vi "3D Plot and Log File Trial1.vi"() -> ()   [LabVIEW 2013]
doc: "This example shows how to use the driver's VI's to set up the Polaris and acquire transformations. For this example, all wired tools are activated and one wireless tool is activated."
uses:
  <vilib>/Platform/NI_3dgraph.lvlib
panel:
  in  "Output File":path=path "c:/polaris.txt"
  in  "STOP 2":bool
  in  "Track Outside Measurement Volume? (F:No) 2":bool
  in  "Track Stray Markers? (F:No)":bool
  out "Current Transformations 2":T1(array[cluster])
  in  "Location of ROM File for Tool":path=path "C:/Program Files/Northern Digital Inc/8700248.rom"
  in  "Serial Configuration":T2={"Baud Rate (9600)"=9600, "Flow Control (0:None)"=0, "Parity"=0, "Data Bits"=8, "Stop Bits"=10} {"Stop Bits" items=["1.0"=10, "2.0"=20]; "Parity" items=["None", "Odd", "Even"]; "Flow Control (0:None)" items=["None", "XON/XOFF"]; "Baud Rate (9600)" items=["9600"=9600, "14.4k"=14400, "19.2k"=19200, "38.4k"=38400, "57.6k "=57600, "115.2k"=115200]}
  out "Current Transformations":T1(array[cluster])
  in  "VISA resource name":refnum<visa-resource-name>="COM1"
  in  "Reset? (T:Yes)":bool=TRUE
  in  "3D Curve":refnum<k7>(container)
  in  "Track Outside Measurement Volume? (F:No)":bool
  in  "Plot Data? (T:Yes)":bool=TRUE
  in  "STOP":bool
  # "NOTE: This VI will only run on machines using a Windows OS (for ActiveX support).  Plotting this 3D data\nis NOT meant for performance, rather it is intended to give a more intuitive representation of the data\nreturned by the Polaris instrument.  For demonstration of faster acquisition, please take a look at the\nndipolaris Measurement Exampole VI."
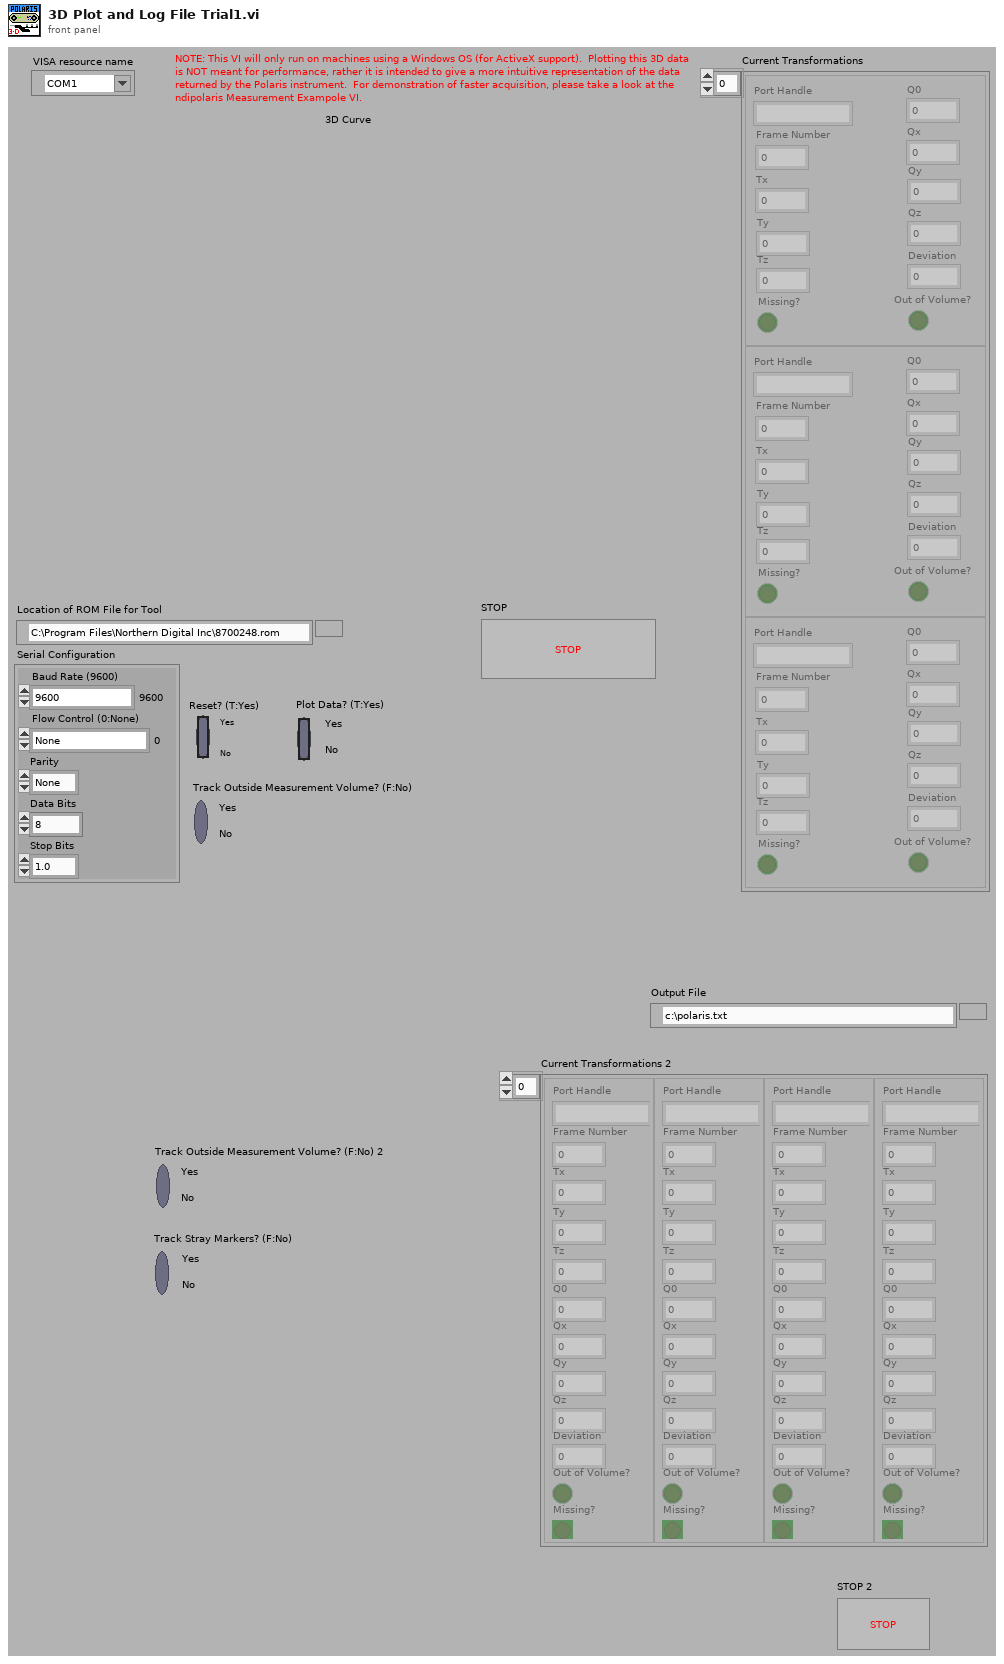
[diagram p1: front panel]
types:
  T1 = cluster{"Port Handle":string, "Frame Number":u32, "Tx":dbl, "Ty":dbl, "Tz":dbl, "Q0":dbl, "Qx":dbl, "Qy":dbl, "Qz":dbl, "Deviation":dbl, "Missing?":bool, "Out of Volume?":bool}[]
  T2 = cluster{"Baud Rate (9600)":u32, "Flow Control (0:None)":u16, "Parity":u16, "Data Bits":u16, "Stop Bits":u16}
  T3 = enum16{"open", "open or create", "create or replace", "create", "open (read only)"}
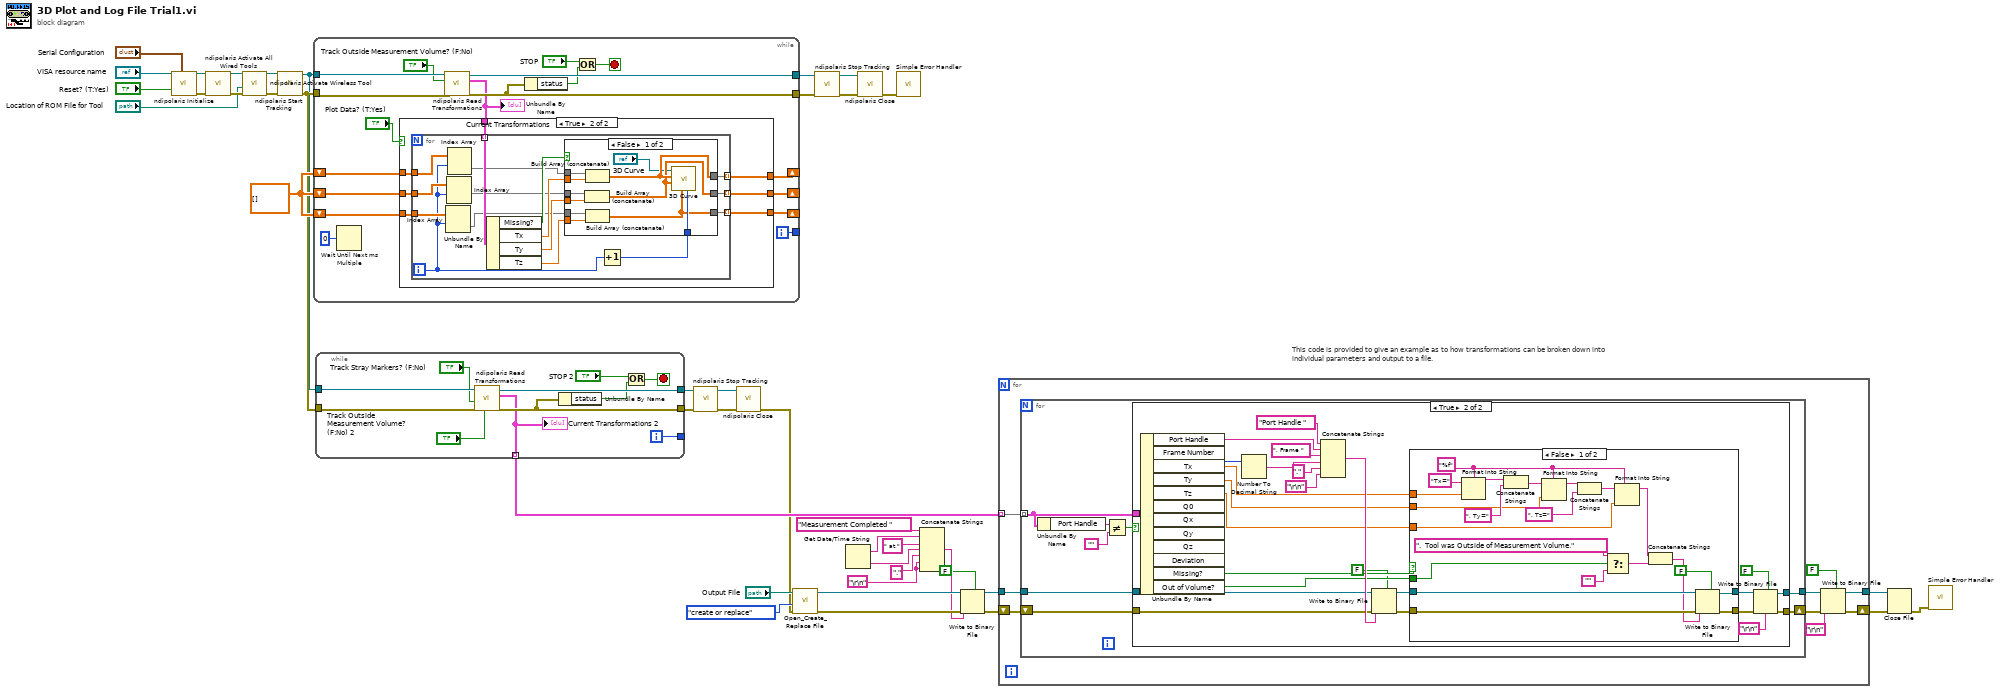
[diagram p0: block diagram]
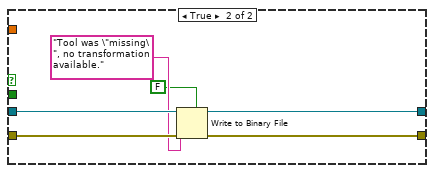
[diagram p3: hidden frame]
diagram:
  w6 = "\r\n"
  w34 = dbl[][] []
  # "This code is provided to give an example as to how transformations can be broken down into\nindividual parameters and output to a file."
  n1 = call <instrlib>:"ndipolaris Initialize.vi"("Serial Configuration"="Serial Configuration", "Reset? (T: Yes)"="Reset? (T:Yes)", "VISA resource name"="VISA resource name") -> ("error out"=w35:errorcluster, "VISA resource name out"=w36:refnum<visa-resource-name>)  [unwired: 7 in]
  n2 = call <instrlib>:"ndipolaris Activate All Wired Tools.vi"("error in (no error)"=w35, "VISA resource name"=w36) -> ("error out"=w39:errorcluster, "VISA resource out"=w40:refnum<visa-resource-name>)  [unwired: 7 in, 1 out]
  n3 = call <instrlib>:"ndipolaris Activate Wireless Tool.vi"("error in (no error)"=w39, "Location of ROM File for Tool"="Location of ROM File for Tool", "VISA resource name"=w40) -> ("error out"=w37:errorcluster, "VISA resource out"=w38:refnum<visa-resource-name>)  [unwired: 6 in, 1 out]
  n4 = call <instrlib>:"ndipolaris Start Tracking.vi"("error in (no error)"=w37, "VISA resource name"=w38) -> ("error out"=w2:errorcluster, "VISA resource out"=w1:refnum<visa-resource-name>)  [unwired: 8 in]
  n5 = while {
    tunnel: w1 -> [w59]
    tunnel: w2 -> [w58]
    tunnel: [w43] -> _
    tunnel: [w53] -> w29
    tunnel: [w52] -> w28
    shift-right: [w46] -> _
    shift-left: w34 -> [w49]
    shift-right: [w45] -> _
    shift-left: w34 -> [w48]
    shift-right: [w44] -> _
    shift-left: w34 -> [w47]
    i -> [w43]
    stop <- w56 stop-if-true
    n6 = Wait Until Next ms Multiple(millisecond multiple=u32 0) -> ()  [unwired: 1 out]
    n7 = call <instrlib>:"ndipolaris Read Transformations.vi"("error in (no error)"=w58, "Get Extended Tool Info? (F:No)"="Track Outside Measurement Volume? (F:No)", "VISA resource name"=w59) -> ("error out"=w52:errorcluster, "Transformations"=w42:T1, "VISA resource out"=w53:refnum<visa-resource-name>)  [unwired: 5 in, 1 out]
    "Current Transformations" <- w42
    n8 = case shown="True" "Plot Data? (T:Yes)" {
      tunnel: w42 -> [_ w69]
      tunnel: w49 -> [w62 w65]
      tunnel: w48 -> [w61 w64]
      tunnel: w47 -> [w60 w63]
      tunnel: [w62 w68] -> w46
      tunnel: [w61 w67] -> w45
      tunnel: [w60 w66] -> w44
      frame False {
      }
      frame True {
        n9 = for {
          tunnel: w69 -> [w85] mode=indexing
          tunnel: [w79] -> w66 mode=indexing
          tunnel: [w78] -> w67 mode=indexing
          tunnel: [w77] -> w68 mode=indexing
          tunnel: w65 -> [w76]
          tunnel: w64 -> [w74]
          tunnel: w63 -> [w75]
          i -> [w73]
          n10 = Index Array(array=w75, index (row)=w73) -> (element=w70:dbl[])  [unwired: 1 in]
          n11 = Index Array(array=w74, index (row)=w73) -> (element=w71:dbl[])  [unwired: 1 in]
          n12 = Index Array(array=w76, index (row)=w73) -> (element=w72:dbl[])  [unwired: 1 in]
          n13 = Unbundle By Name(w85) -> ("Missing?"=w84:bool, "Tx"=w83:dbl, "Ty"=w82:dbl, "Tz"=w81:dbl)
          n14 = Increment(x=w73) -> (x+1=w80:i32)
          n15 = case shown="False" w84 {
            tunnel: w83 -> [w96 _]
            tunnel: w82 -> [w95 _]
            tunnel: w81 -> [w94 _]
            tunnel: w80 -> [w93 _]
            tunnel: [w92 w99] -> w77
            tunnel: [w91 w98] -> w78
            tunnel: [w90 w97] -> w79
            tunnel: w72 -> [w89 w99]
            tunnel: w71 -> [w88 w98]
            tunnel: w70 -> [w87 w97]
            frame False {
              n16 = Build Array (concatenate)(w88, w95) -> (w91:dbl[])
              n17 = Build Array (concatenate)(w89, w96) -> (w92:dbl[])
              n18 = Build Array (concatenate)(w87, w94) -> (w90:dbl[])
              n19 = call <vilib>:"3D Curve.vi"("plot number (1)"=w93, "z vector"=w90, "y vector"=w91, "x vector"=w92, "3D graph"="3D Curve") -> ()  [unwired: 5 in, 2 out]
            }
            frame True {
            }
          }
        }
      }
    }
    n20 = Unbundle By Name(w52) -> ("status"=w51:bool)
    n21 = Or(x="STOP", y=w51) -> (x .or. y?=w56:bool)
  }
  n22 = while {
    tunnel: w1 -> [w110]
    tunnel: w2 -> [w109]
    tunnel: [w103] -> _
    tunnel: [w106] -> w25
    tunnel: [w105] -> w24
    tunnel: [w100] -> w21 mode=indexing
    i -> [w103]
    stop <- w108 stop-if-true
    n23 = call <instrlib>:"ndipolaris Read Transformations.vi"("Track Outside Measurement Volume? (F:No)"="Track Outside Measurement Volume? (F:No) 2", "error in (no error)"=w109, "Track Stray Markers? (F:No)"="Track Stray Markers? (F:No)", "VISA resource name"=w110) -> ("error out"=w105:errorcluster, "Transformations"=w100:T1, "VISA resource out"=w106:refnum<visa-resource-name>)  [unwired: 4 in, 1 out]
    "Current Transformations 2" <- w100
    n24 = Unbundle By Name(w105) -> ("status"=w104:bool)
    n25 = Or(x="STOP 2", y=w104) -> (x .or. y?=w108:bool)
  }
  n26 = call <instrlib>:"ndipolaris Stop Tracking.vi"("error in (no error)"=w24, "VISA resource name"=w25) -> ("error out"=w22:errorcluster, "VISA resource out"=w23:refnum<visa-resource-name>)  [unwired: 8 in]
  n27 = call <instrlib>:"ndipolaris Close.vi"("error in (no error)"=w22, "VISA resource name"=w23) -> ("error out"=w5:errorcluster)  [unwired: 9 in]
  n28 = call <vilib>:"Open_Create_Replace File.vi"("error in (no error)"=w5, "function (open:0)"=T3."create or replace", "file path"="Output File") -> ("error out"=w17:errorcluster, "refnum"=w18:refnum<file>)  [unwired: 5 in, 2 out]
  n29 = call <instrlib>:"ndipolaris Stop Tracking.vi"("error in (no error)"=w28, "VISA resource name"=w29) -> ("error out"=w31:errorcluster, "VISA resource out"=w32:refnum<visa-resource-name>)  [unwired: 8 in]
  n30 = Get Date/Time String() -> (date string=w15:string, time string=w13:string)  [unwired: 3 in]
  n31 = call <instrlib>:"ndipolaris Close.vi"("error in (no error)"=w31, "VISA resource name"=w32) -> ("error out"=w30:errorcluster)  [unwired: 9 in]
  n32 = call <vilib>:"Simple Error Handler.vi"("error in (no error)"=w30) -> ()  [unwired: 4 in, 5 out]
  n33 = Concatenate Strings("Measurement Completed ", w15, " at ", w13, "." ("string"), w6, w6) -> (w12:string)
  n34 = Write to Binary File(file (use dialog)=w18, data=w12, error in=w17, 5:FALSE ("prepend array or string size? (T)")) -> (refnum out=w11:refnum<file>, error out=w10:errorcluster)  [unwired: 2 in, 1 out]
  n35 = for {
    tunnel: w21 -> [w119] mode=indexing
    tunnel: w11 -> [w118]
    shift-right: [w113] -> w8
    shift-left: w10 -> [w117]
    tunnel: [w114] -> w9
    n36 = for {
      tunnel: w119 -> [w123] mode=indexing
      tunnel: w118 -> [w127]
      tunnel: [w125] -> w115
      shift-right: [w124] -> w116
      shift-left: w117 -> [w126]
      n37 = Unbundle By Name(w123) -> ("Port Handle"=w122:string)
      n38 = Not Equal?(x=w122, y="") -> (x != y?=w121:bool)
      n39 = case shown="True" w121 {
        tunnel: w123 -> [_ w154]
        tunnel: w127 -> [w129 w146]
        tunnel: w126 -> [w128 w145]
        tunnel: [w129 w135] -> w125
        tunnel: [w128 w134] -> w124
        frame False {
        }
        frame True {
          n40 = Unbundle By Name(w154) -> ("Port Handle"=w148:string, "Frame Number"=w153:u32, "Tx"=w140:dbl, "Ty"=w139:dbl, "Tz"=w138:dbl, "Missing?"=w141:bool, "Out of Volume?"=w132:bool)  [unwired: 5 out]
          n41 = Number To Decimal String(number=w153) -> (decimal integer string=w151:string)  [unwired: 1 in]
          n42 = Concatenate Strings("Port Handle " ("string"), w148, ", Frame ", w151, "." ("string"), "\r\n") -> (w147:string)
          n43 = Write to Binary File(file (use dialog)=w146, data=w147, error in=w145, 5:FALSE ("prepend array or string size? (T)")) -> (refnum out=w143:refnum<file>, error out=w142:errorcluster)  [unwired: 2 in, 1 out]
          n44 = case shown="False" w141 {
            tunnel: w143 -> [w163 w182]
            tunnel: w142 -> [w162 w181]
            tunnel: [w165 w179] -> w136
            tunnel: [w164 w178] -> w137
            tunnel: w140 -> [w175 _]
            tunnel: w139 -> [w171 _]
            tunnel: w138 -> [w166 _]
            tunnel: w132 -> [w159 _]
            frame False {
              w168 = "%f" ("format string")
              n45 = Format Into String(format string=w168, initial string="Tx=", w175) -> (resulting string=w174:string)  [unwired: 1 in, 1 out]
              n46 = Concatenate Strings(w174, ", Ty=") -> (w172:string)
              n47 = Format Into String(format string=w168, initial string=w172, w171) -> (resulting string=w170:string)  [unwired: 1 in, 1 out]
              n48 = Concatenate Strings(w170, ", Tz=") -> (w169:string)
              n49 = Select(t=".  Tool was Outside of Measurement Volume.", s=w159, f="") -> (s? t:f=w156:string)
              n50 = Format Into String(format string=w168, initial string=w169, w166) -> (resulting string=w161:string)  [unwired: 1 in, 1 out]
              n51 = Concatenate Strings(w161, w156) -> (w160:string)
              n52 = Write to Binary File(file (use dialog)=w163, data=w160, error in=w162, 5:FALSE ("prepend array or string size? (T)")) -> (refnum out=w165:refnum<file>, error out=w164:errorcluster)  [unwired: 2 in, 1 out]
            }
            frame True {
              n53 = Write to Binary File(file (use dialog)=w182, data="Tool was \"missing\", no transformation available.", error in=w181, 5:FALSE ("prepend array or string size? (T)")) -> (refnum out=w179:refnum<file>, error out=w178:errorcluster)  [unwired: 2 in, 1 out]
            }
          }
          n54 = Write to Binary File(file (use dialog)=w136, data="\r\n", error in=w137, 5:FALSE ("prepend array or string size? (T)")) -> (refnum out=w135:refnum<file>, error out=w134:errorcluster)  [unwired: 2 in, 1 out]
        }
      }
    }
    n55 = Write to Binary File(file (use dialog)=w115, data="\r\n", error in=w116, 5:FALSE ("prepend array or string size? (T)")) -> (refnum out=w114:refnum<file>, error out=w113:errorcluster)  [unwired: 2 in, 1 out]
  }
  n56 = Close File(refnum=w9, error in=w8) -> (error out=w4:errorcluster)  [unwired: 1 out]
  n57 = call <vilib>:"Simple Error Handler.vi"("error in (no error)"=w4) -> ()  [unwired: 4 in, 5 out]
